vi "Binding Employee Table.vi"(8 "error in (no error)":errorcluster caption="错误输入（无错误）", 10 "Select Table":T1, 11 "Employee 输入":refnum<class "Employee.lvclass"> caption="DNL_LabVIEW Object in") -> (0 "error out":errorcluster caption="错误输出", 3 "Employee 输出":refnum<class "Employee.lvclass"> caption="DNL_LabVIEW Object out")   [LabVIEW 2012, in "Employee.lvclass"]
uses:
  Employee.lvclass
  Custom Def/Select Table.ctl
  Employee.lvclass/Employee.ctl
  Data Set/DataSet.lvclass
  Data Table/DataTable.lvclass
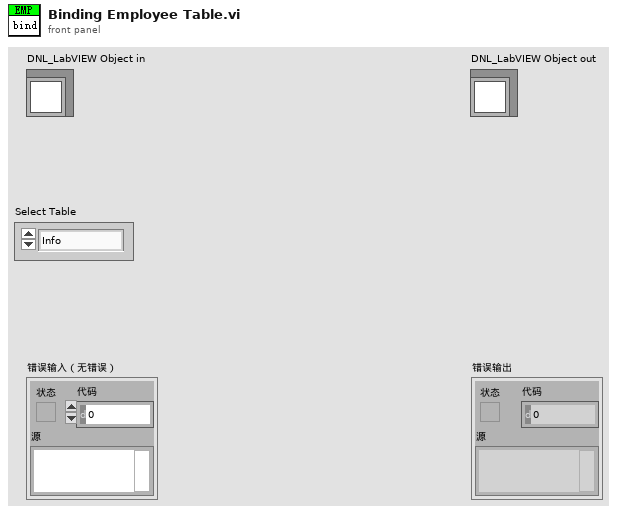
[diagram p1: front panel]
types:
  T1 = typedef "Select Table.ctl" = enum16{"Info", "Salary"}
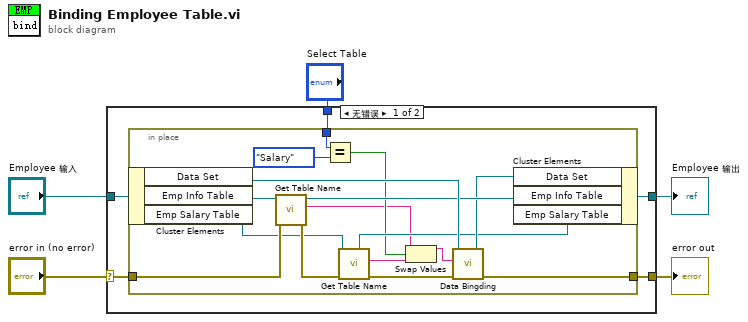
[diagram p0: block diagram]
diagram:
  n1 = case shown="无错误" "error in (no error)" {
    selector: "error in (no error)" -> [w8 w28]
    tunnel: [w9 w28] -> w4
    tunnel: [w7 w27] -> w2
    tunnel: "Employee 输入" -> [w10 w27]
    tunnel: "Select Table" -> [w6 _]
    frame No Error {
      n2 = in-place {
        in-place-border: w8 -> [w24]
        in-place-border: [w21] -> w9
        in-place-border: w6 -> [w16]
        n3 = in-place-cluster #1(w10) -> ("Data Set"=w26:refnum<class "DataSet.lvclass">, "Emp Info Table"=w25:refnum<class "DataTable.lvclass">, "Emp Salary Table"=w19:refnum<class "DataTable.lvclass">)
        n4 = call "Get Table Name.vi"("error in (no error)"=w24, "DataTable输入"=w25) -> ("error out"=w20:errorcluster, "Table Name"=w13:string, "DataTable输出"=w23:refnum<class "DataTable.lvclass">)  [unwired: 7 in]
        n5 = Equal?(x=w16, y=Select_Table."Salary") -> (x = y?=w14:bool)
        n6 = call "Get Table Name.vi"("error in (no error)"=w20, "DataTable输入"=w19) -> ("error out"=w17:errorcluster, "Table Name"=w12:string, "DataTable输出"=w18:refnum<class "DataTable.lvclass">)  [unwired: 7 in]
        n7 = Swap Values(12:w13, 13:w14, 14:w12) -> (1:w11:string)  [unwired: 1 out]
        n8 = call "Data Bingding.vi"("error in (no error)"=w17, "dataMember"=w11, "DataSet 输入"=w26) -> ("error out"=w21:errorcluster, "DataSet 输出"=w22:refnum<class "DataSet.lvclass">)  [unwired: 7 in]
        n9 = in-place-cluster #1("Data Set"=w22, "Emp Info Table"=w23, "Emp Salary Table"=w18) -> (w7:refnum<class "Employee.lvclass">)
      }
    }
    frame Error {
    }
  }
  "error out" <- w4
  "Employee 输出" <- w2
